vi "Add Sequence Element.vi"(8 "error in (no error)":errorcluster, 10 "Name":string, 11 "Sequence Controller in":refnum<class "Sequence Controller.lvclass">) -> (0 "error out":errorcluster, 3 "Sequence Controller out":refnum<class "Sequence Controller.lvclass">)   [LabVIEW 2016, in "Sequence Controller.lvclass"]
uses:
  Sequence Controller.lvclass
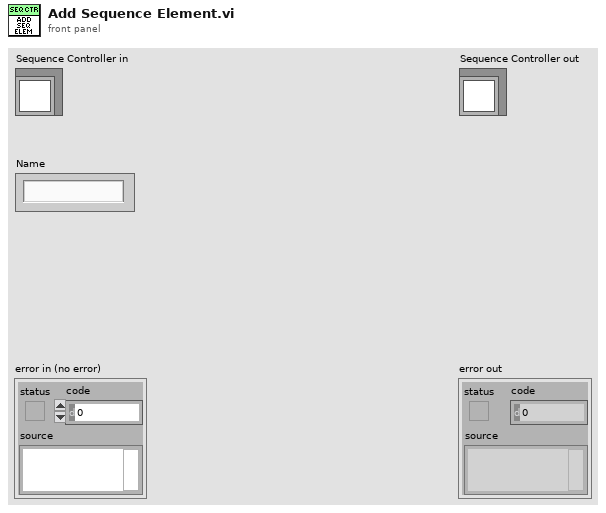
[diagram p1: front panel]
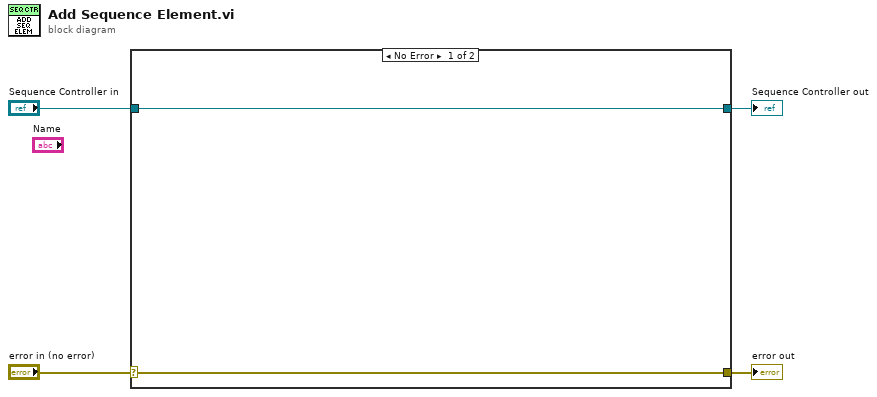
[diagram p0: block diagram]
diagram:
  n1 = case shown="No Error" "error in (no error)" {
    selector: "error in (no error)" -> [w5 w8]
    tunnel: [w5 w8] -> w3
    tunnel: [w6 w7] -> w1
    tunnel: "Sequence Controller in" -> [w6 w7]
    frame No Error {
    }
    frame Error {
    }
  }
  "error out" <- w3
  "Sequence Controller out" <- w1
